vi "BRig_dataCurrent_LaserSwitch_l2.vi"() -> (2 "output_LaserSwitch_l2":i32)   [LabVIEW 2014]
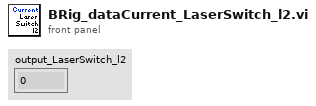
[diagram p1: front panel]
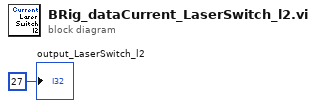
[diagram p0: block diagram]
diagram:
  "output_LaserSwitch_l2" <- 27 ("output_iBlock")
